vi "SavePath.vi"(11 "字符串":string) -> (3 "appended path":path)   [LabVIEW 2014, in "ChaxuConfig.lvlib"]
uses:
  ChaxuConfig.lvlib
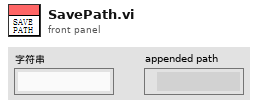
[diagram p1: front panel]
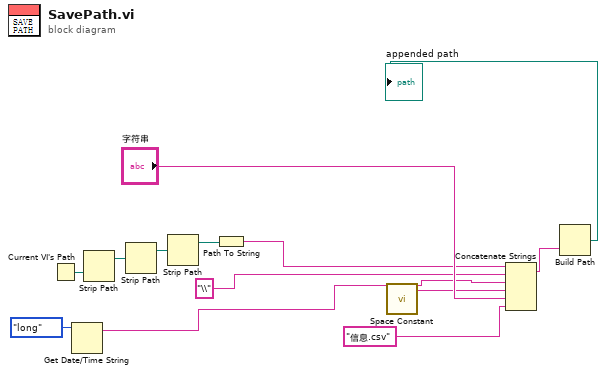
[diagram p0: block diagram]
diagram:
  n1 = Current VI's Path() -> (path=w1:path)
  n2 = Get Date/Time String(date format (0)=enum16{"short", "long", "abbreviated"}."long" ("日期格式(0)")) -> (date string=w9:string)  [unwired: 2 in, 1 out]
  n3 = Strip Path(path=w1) -> (stripped path=w2:path)  [unwired: 1 out]
  n4 = Strip Path(path=w2) -> (stripped path=w4:path)  [unwired: 1 out]
  n5 = Strip Path(path=w4) -> (stripped path=w5:path)  [unwired: 1 out]
  n6 = Path To String(path=w5) -> (string=w6:string)
  n7 = call <vilib>:"Space Constant.vi"() -> ("String"=w8:string)
  n8 = Concatenate Strings(w6, "\\", w9, w8, "字符串", "信息.csv") -> (w7:string)
  n9 = Build Path(name or relative path=w7) -> (appended path=→"appended path":path)  [unwired: 1 in]
